vi "Analysis-Complete.vi"(8 "error in (no error)":errorcluster, 9 "selected path":path, 10 "VI reference":refnum<vi>) -> (0 "error out":errorcluster, 1 "File Path Out":path, 2 "PTP Array":dbl[](array[numeric]), 3 "SGP Array":dbl[](array[numeric]), 5 "error?":bool)   [LabVIEW 2020]
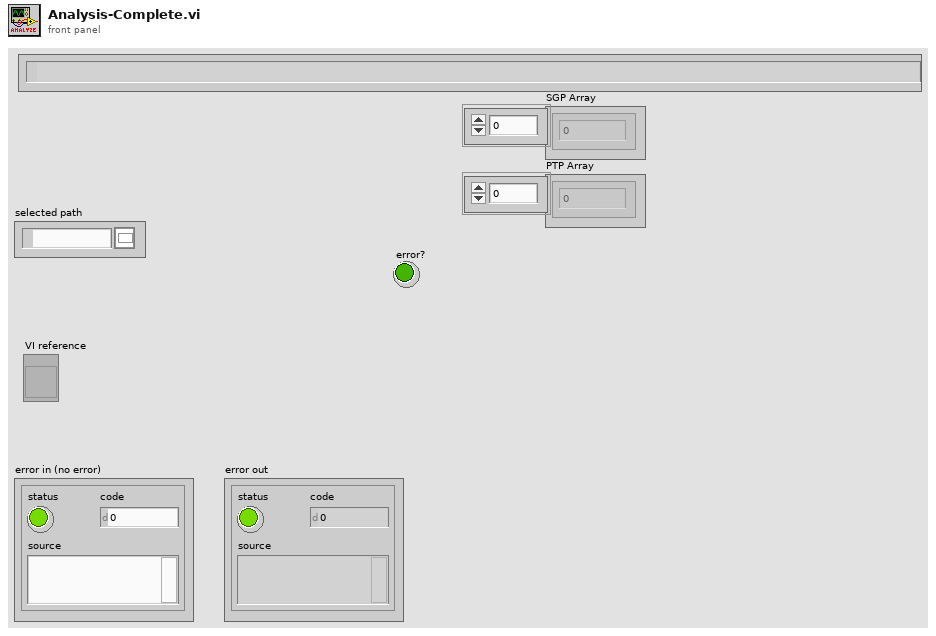
[diagram p1: front panel]
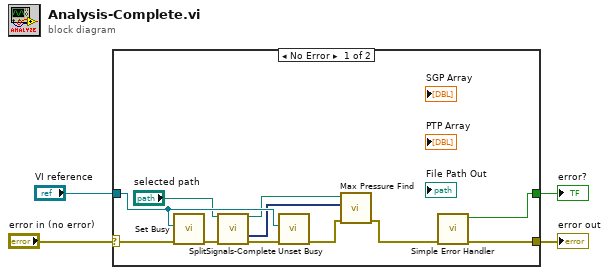
[diagram p0: block diagram]
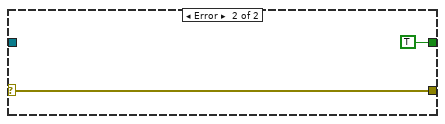
[diagram p2: hidden frame]
diagram:
  n1 = case shown="No Error" "error in (no error)" {
    selector: "error in (no error)" -> [w15 w17]
    tunnel: [w13 w17] -> w4
    tunnel: "VI reference" -> [w14 _]
    tunnel: [w12 TRUE ("error?")] -> w1
    frame No Error {
      n2 = call <vilib>:"Set Busy.vi"("error in (no error)"=w15, "VI reference (current VI)"=w14) -> ("error out"=w10:errorcluster)  [unwired: 8 in, 1 out]
      n3 = call "SplitSignals-Complete.vi"("Filename"="selected path", "Error In"=w10) -> ("Filename Out"=w6:path, "Pressure"=w5:dynamicdata, "Error Out"=w11:errorcluster)  [unwired: 10 in, 1 out]
      n4 = call <vilib>:"Unset Busy.vi"("error in (no error)"=w11, "VI reference (current VI)"=w14) -> ("error out"=w8:errorcluster)  [unwired: 9 in]
      n5 = call "Max Pressure Find.vi"("Error In"=w8, "Pressure"=w5, "File Path"=w6) -> ("Error Out"=w7:errorcluster)  [unwired: 6 in, 2 out]
      n6 = call <vilib>:"Simple Error Handler.vi"("error in (no error)"=w7) -> ("error?"=w12:bool, "error out"=w13:errorcluster)  [unwired: 4 in, 3 out]
    }
    frame Error {
    }
  }
  "error out" <- w4
  "error?" <- w1
